vi "S2C_OM8257_Proc_SendCmd.vi"(7 "Local?":bool, 8 "Error In":errorcluster, 10 "Command":string, 11 "JSON String":string) -> (0 "Error Out":errorcluster, 3 "Response":variant)   [LabVIEW 2015]
uses:
  Uni-Therm/VIs/S2C_UNITHERM_Proc_Globals.vi
  S2C_OM8257_Proc_Globals.vi
  <instrlib>/Associated Research 82XX/Associated Research 82XX.lvlib
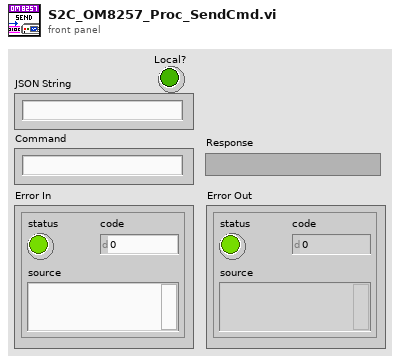
[diagram p1: front panel]
types:
  T1 = cluster{"Voltage (V)":u16, "High Limit Total (mA)":dbl, "Low Limit Total (mA)":dbl, "Ramp Up Time (s)":dbl, "Dwell Time (s)":dbl, "Arc Sense":u8, "Arc Detect":bool, "High Limit Real (mA)":dbl, "Low Limit Real (mA)":dbl, "Ramp Down Time (s)":dbl, "Continuity":bool, "Offset (mA)":dbl, "Auto Offset":bool, "DUT Output":bool, "Frequency (Hz)":u16, "Scanner?":bool, "Step Selection":i32, "Add Step":bool, "Scan1":i32, "Scan2":i32, "Scan3":i32, "Scan4":i32, "Scan5":i32, "Scan6":i32, "Scan7":i32, "Scan8":i32, "Scan9":i32, "Scan10":i32, "Scan11":i32, "Scan12":i32, "Scan13":i32, "Scan14":i32, "Scan15":i32, "Scan16":i32}
  T2 = cluster{"Scan1":i32, "Scan2":i32, "Scan3":i32, "Scan4":i32, "Scan5":i32, "Scan6":i32, "Scan7":i32, "Scan8":i32, "Scan9":i32, "Scan10":i32, "Scan11":i32, "Scan12":i32, "Scan13":i32, "Scan14":i32, "Scan15":i32, "Scan16":i32}
  T3 = cluster{"Voltage (1240V)":u16, "High Limit Total (10mA)":dbl, "Low Limit Total (0mA)":dbl, "Ramp Up Time (0.1s)":dbl, "Dwell Time (1s)":dbl, "Arc Sense (5)":u8, "Arc Detect (F: Off)":bool, "High Limit Real(10mA)":dbl, "Low Limit Real (0mA)":dbl, "Ramp Down Time (1s)":dbl, "Continuity (F: Off)":bool, "Offset (0mA)":dbl, "Auto Offset (F: Off)":bool, "DUT Output (F: Off)":bool, "Frequency (60Hz)":u16}
  T4 = cluster{"Leakage-Hi (V)":dbl, "Leakage-Lo (V)":dbl, "Voltage-Hi (V)":dbl, "Voltage-Lo (V)":dbl, "Dwell (s)":dbl, "Delay (s)":dbl, "Offset (uA)":dbl, "AC Src Voltage (V)":dbl, "AC Src A-Hi (A)":dbl, "AC Source":bool, "AC Src Frequency":dbl, "Auto Offset":bool, "Reverse":bool, "Active Link":bool, "AC Src OC Fold":bool, "Neutral":bool, "Ground":bool, "Leakage":bool, "Ranging Mode":bool, "AC Src Output":bool, "AC Src Range":bool, "Measure Device":u16, "Probe":u16, "Filter Mode":u16, "Scanner?":bool, "Step Selection":i32, "Add Step":bool, "Scan1":i32, "Scan2":i32, "Scan3":i32, "Scan4":i32, "Scan5":i32, "Scan6":i32, "Scan7":i32, "Scan8":i32, "Scan9":i32, "Scan10":i32, "Scan11":i32, "Scan12":i32, "Scan13":i32, "Scan14":i32, "Scan15":i32, "Scan16":i32}
  T5 = cluster{"Leakage-Hi (6000V)":dbl, "Leakage-Lo (0uA)":dbl, "Voltage-Hi (125V)":dbl, "Voltage-Lo (0V)":dbl, "Dwell (0.5s)":dbl, "Delay (1s)":dbl, "Offset  (0uA)":dbl, "AC Source Voltage (115V)":dbl, "AC Source A-Hi (0A)":dbl, "AC Source (F: OFF)":bool, "AC Source Frequency (60Hz)":dbl, "Auto Offset (F:OFF)":bool, "Reverse (F:OFF)":bool, "Active Link (F:OFF)":bool, "AC Source OC Fold (F:OFF)":bool, "Neutral (F:CLOSED)":bool, "Ground (F:CLOSED)":bool, "Leakage (F:RMS)":bool, "Ranging Mode (Auto)":bool, "AC Source Output (T:OPEN)":bool, "AC Source Range (F:LOW)":bool, "Measure Device (UL544NP)":u16, "Probe (Ground TO Line)":u16, "Filter Mode (AC+DC)":u16}
  T6 = cluster{"Current (25A)":dbl, "Voltage (8V)":dbl, "Hi-Limit (100mohm)":u16, "Lo-Limit (0mohm)":u16, "Dwell (1s)":dbl, "Offset (0mohm)":u16, "Auto Offset (OFF)":bool, "Frequency (60Hz)":u16, "DualCHEK (OFF)":u16}
  T7 = cluster{"Current (A)":dbl, "Voltage (V)":dbl, "Hi-Limit (mohm)":u16, "Lo-Limit (mhom)":u16, "Dwell (s)":dbl, "Offset (mhom)":u16, "Auto Offset":bool, "Frequency (Hz)":u16, "DualCHEK":u16, "Scanner Selection":i32, "Scanner?":bool, "Step Selection":i32, "Add Step":bool}
  T8 = cluster{"Voltage-Hi (125V)":dbl, "Voltage-Lo (0V)":dbl, "Amp-Hi (10A)":dbl, "Amp-Lo (0A)":dbl, "Dwell (1s)":dbl, "Delay (0.2s)":dbl, "Leakag-Hi (10mA)":dbl, "Leakage-Lo (0mA)":dbl, "Power-Hi (1000W)":u16, "Power-Lo (0W)":u16, "PF-Hi (1)":dbl, "PF-Lo (0)":dbl, "AC Source Voltage (115V)":dbl, "AC Source A-Hi (0A)":dbl, "AC Source (F: OFF)":bool, "AC Source Frequency (60Hz)":u16, "AC Source OC Fold (F:OFF)":bool, "AC Source Output (T:OPEN)":bool, "AC Source Range (F:LOW)":bool, "Active Link (F:OFF)":bool}
  T9 = cluster{"Voltage-Hi (V)":dbl, "Voltage-Lo (V)":dbl, "Amp-Hi (A)":dbl, "Amp-Lo (A)":dbl, "Dwell (s)":dbl, "Delay (s)":dbl, "Leakage-Hi (mA)":dbl, "Leakage-Lo (mA)":dbl, "Power-Hi (W)":u16, "Power-Lo (W)":u16, "PF-Lo":dbl, "PF-Hi":dbl, "AC Src Voltage (V)":dbl, "AC Src A-Hi (A)":dbl, "AC Source":bool, "AC Src Frequency (Hz)":u16, "AC Src OC Fold":bool, "AC Src Output":bool, "AC Src Range":bool, "Active Link":bool, "Step Selection":i32, "Add Step":bool}
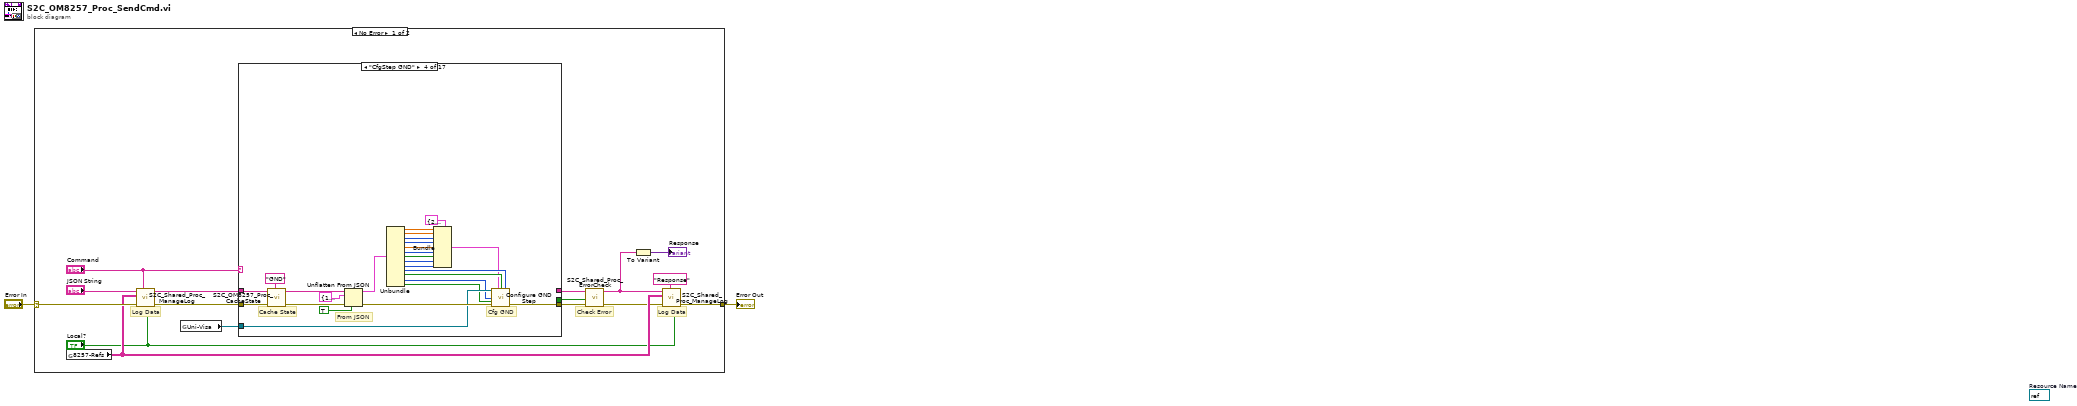
[diagram p0: block diagram]
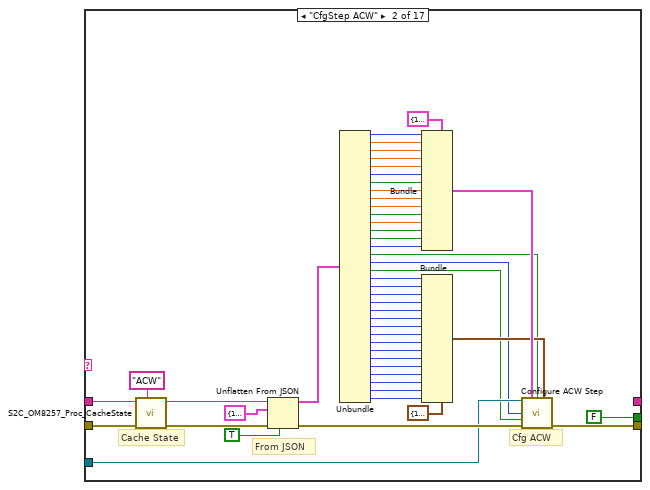
[diagram p3: hidden frame]
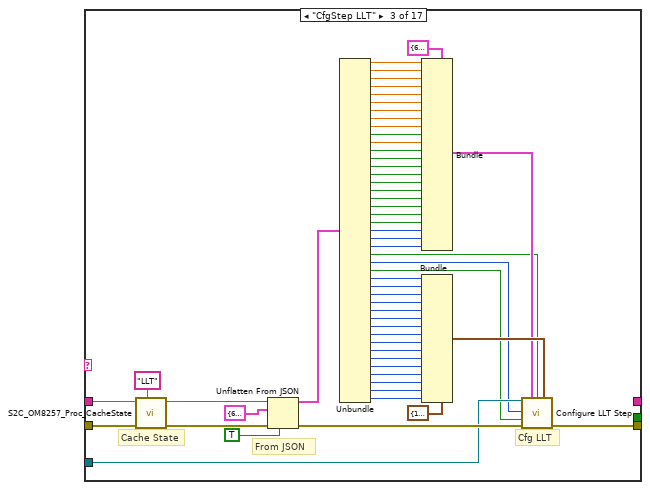
[diagram p4: hidden frame]
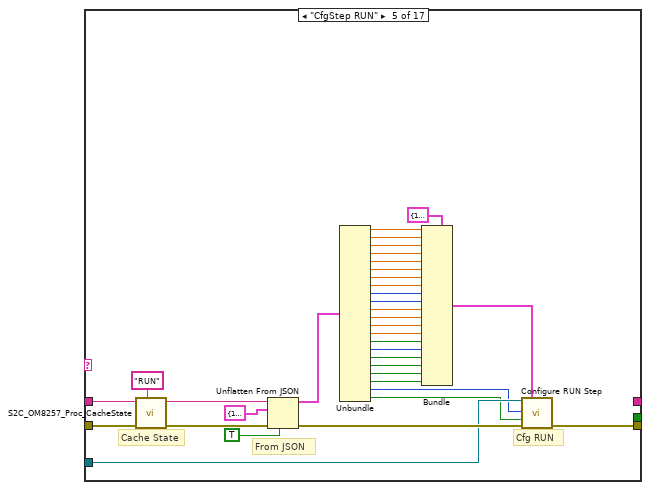
[diagram p5: hidden frame]
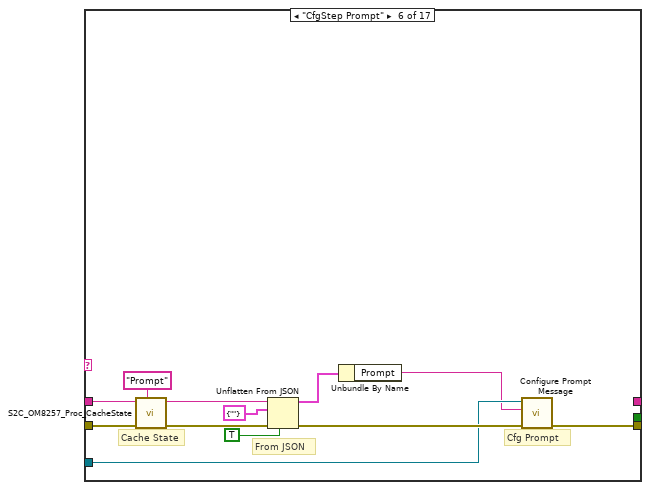
[diagram p6: hidden frame]
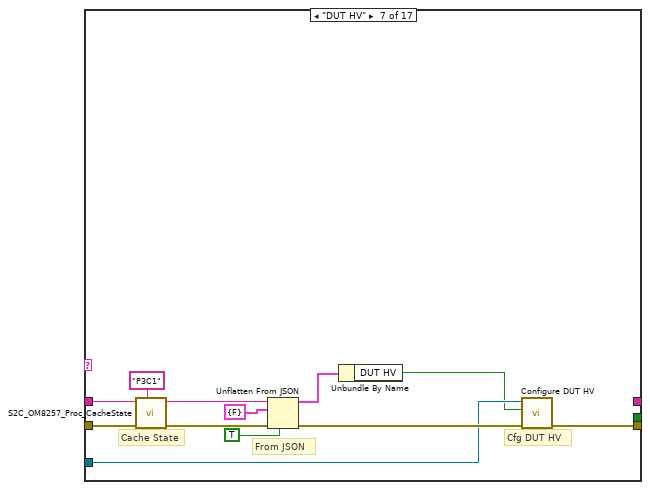
[diagram p7: hidden frame]
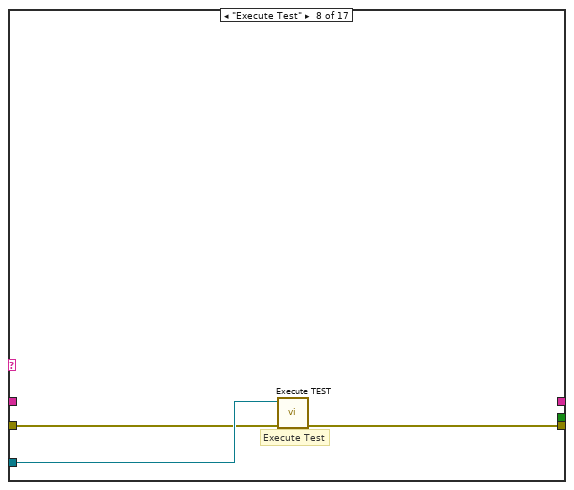
[diagram p8: hidden frame]
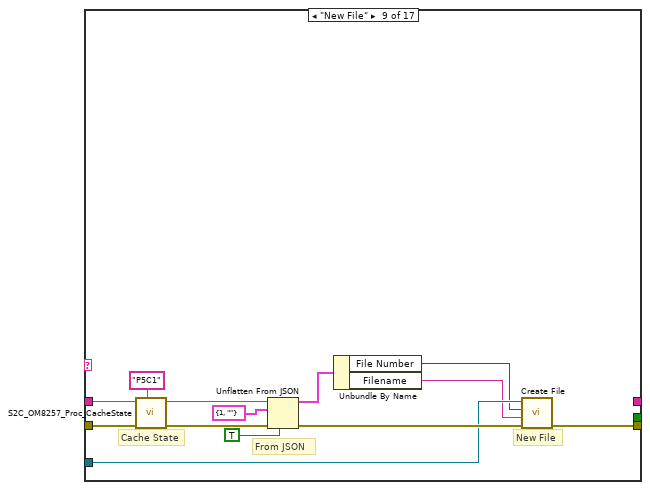
[diagram p9: hidden frame]
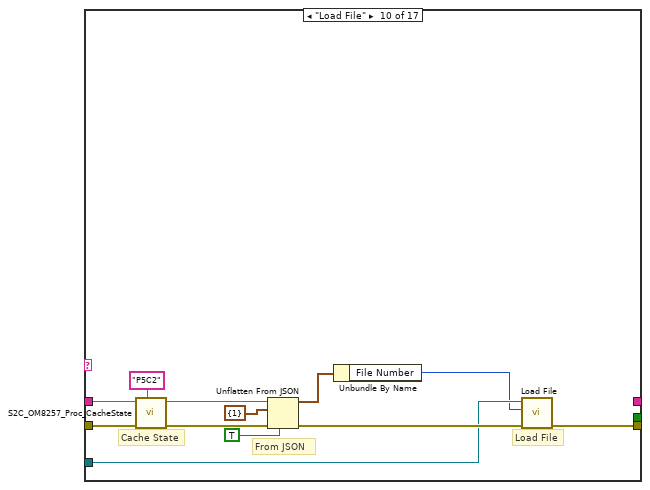
[diagram p10: hidden frame]
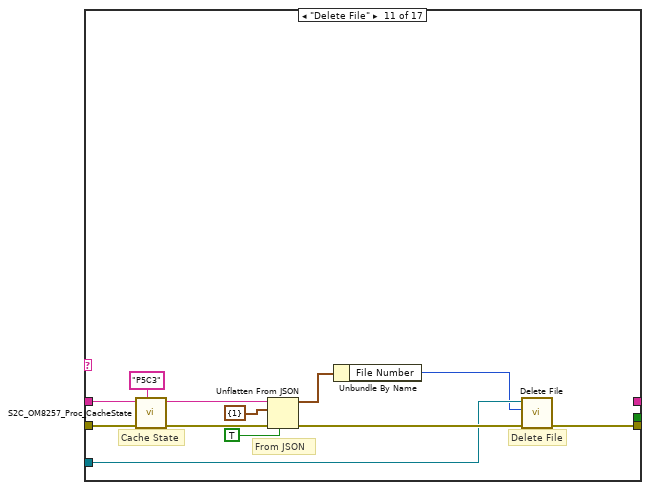
[diagram p11: hidden frame]
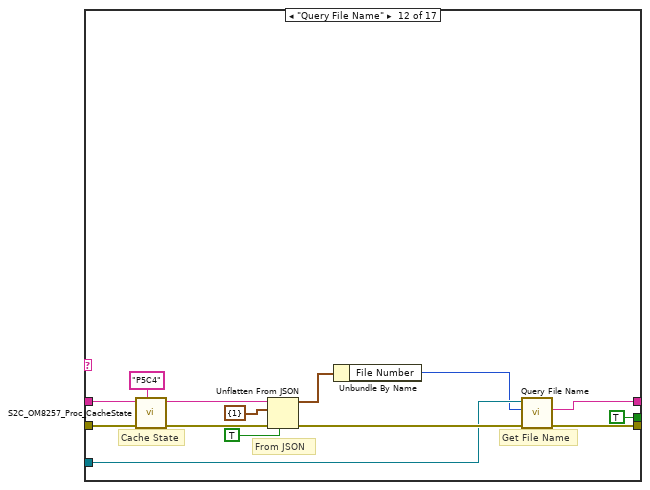
[diagram p12: hidden frame]
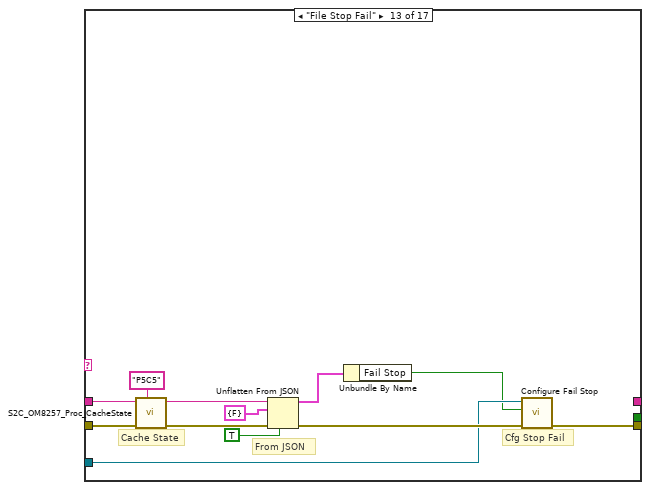
[diagram p13: hidden frame]
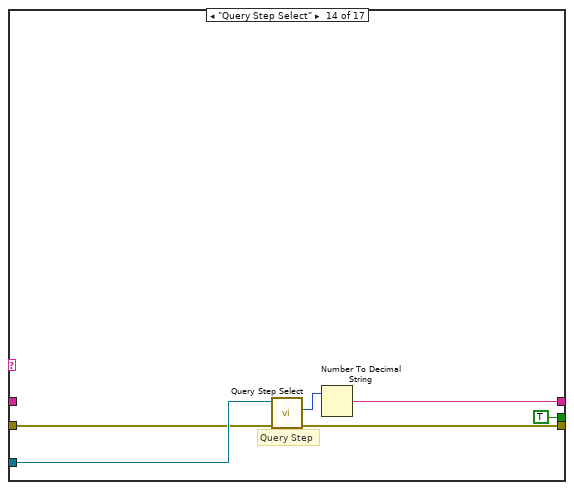
[diagram p14: hidden frame]
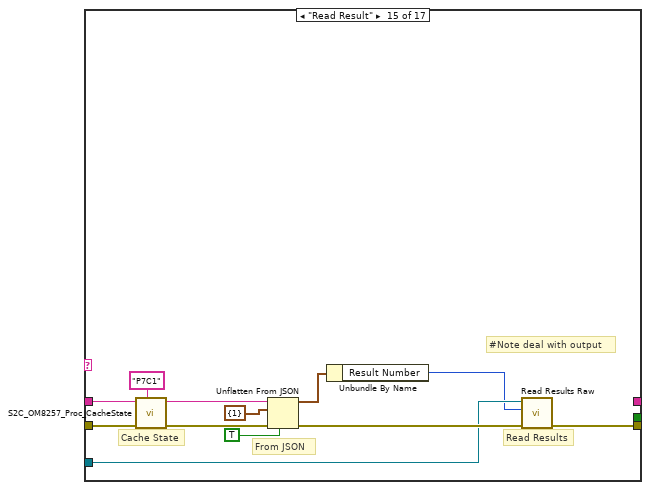
[diagram p15: hidden frame]
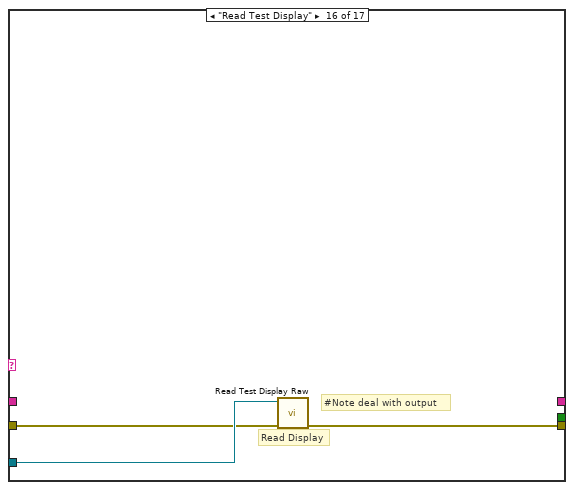
[diagram p16: hidden frame]
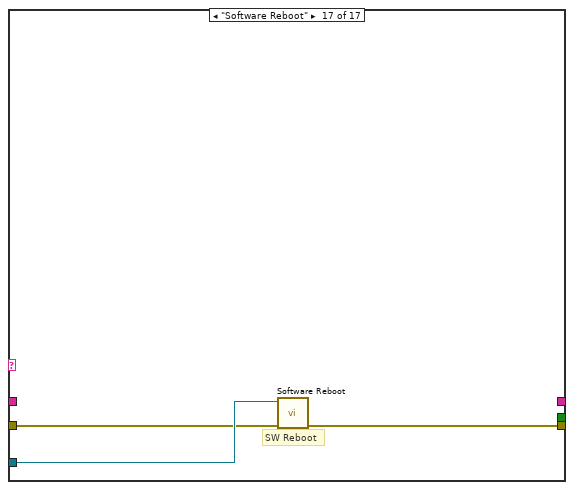
[diagram p17: hidden frame]
diagram:
  (unwired) refnum<visa-resource-name> refnum  # Resource Name
  n1 = case shown="No Error" "Error In" {
    selector: "Error In" -> [w17 w303]
    tunnel: [w16 w303] -> w1
    frame No Error {
      # "Check Error"
      # "Log Data"
      # "Log Data"
      n2 = global read "S2C_OM8257_Proc_Globals.vi" "8257-Refs"() -> (w14:string[][])
      n3 = call "S2C_Shared_Proc_ManageLog.vi"("Local?"="Local?", "Command"="Command", "Error In"=w17, "Refs"=w14, "Data In"="JSON String") -> ("Error Out"=w8:errorcluster, "Data Out"=w7:string)  [unwired: 5 in]
      n4 = global read "S2C_UNITHERM_Proc_Globals.vi" "Uni-Visa"() -> (w6:refnum<visa-resource-name>)
      n5 = case shown="\"CfgStep GND\"" "Command" {
        tunnel: [w19 w67 w125 w151 w186 w198 w210 w215 w226 w238 w250 w264 w276 w284 w294 w299 w302] -> w13
        tunnel: w8 -> [w19 w65 w123 w149 w184 w196 w208 w213 w224 w236 w248 w262 w274 w282 w292 w297 w300]
        tunnel: w7 -> [_ w64 w122 w148 w183 w195 w207 _ w223 w235 w247 w261 w273 _ w291 _ _]
        tunnel: w6 -> [_ w59 w119 w145 w180 w192 w204 w214 w220 w232 w244 w258 w270 w283 w288 w298 w301]
        tunnel: [_ FALSE ("ExpReply?") _ _ _ _ _ _ _ _ _ TRUE ("ExpReply?") _ TRUE ("ExpReply?") _ _ _] -> w5
        tunnel: [_ _ _ _ _ _ _ _ _ _ _ w254 _ w281 _ _ _] -> w3
        frame "Other", Default {
        }
        frame "CfgStep ACW" {
          # "Cache State"
          # "Cfg ACW"
          # "From JSON"
          n6 = call "S2C_OM8257_Proc_CacheState.vi"("Label"="ACW", "Error In"=w65, "Data In"=w64) -> ("Error Out"=w63:errorcluster, "Data Out"=w62:string)  [unwired: 7 in]
          n7 = Unflatten From JSON(JSON string=w62, type and defaults=T1 {"Voltage (V)"=1240, "High Limit Total (mA)"=10.0, "Low Limit Total (mA)"=0.0, "Ramp Up Time (s)"=0.1, "Dwell Time (s)"=1.0, "Arc Sense"=5, "Arc Detect"=FALSE, "High Limit Real (mA)"=10.0, "Low Limit Real (mA)"=0.0, "Ramp Down Time (s)"=0.0, "Continuity"=FALSE, "Offset (mA)"=0.0, "Auto Offset"=FALSE, "DUT Output"=FALSE, "Frequency (Hz)"=60, "Scanner?"=FALSE, "Step Selection"=1, "Add Step"=FALSE, "Scan1"=1, "Scan2"=1, "Scan3"=1, "Scan4"=1, "Scan5"=1, "Scan6"=1, "Scan7"=1, "Scan8"=1, "Scan9"=1, "Scan10"=1, "Scan11"=1, "Scan12"=1, "Scan13"=1, "Scan14"=1, "Scan15"=1, "Scan16"=1} ("ACW"), default null elements? (F)=TRUE, error in (no error)=w63) -> (value=w39:T1, error out=w68:errorcluster)  [unwired: 3 in]
          n8 = Unbundle(w39) -> ("Voltage (V)"=w34:u16, "High Limit Total (mA)"=w33:dbl, "Low Limit Total (mA)"=w32:dbl, "Ramp Up Time (s)"=w31:dbl, "Dwell Time (s)"=w30:dbl, "Arc Sense"=w29:u8, "Arc Detect"=w28:bool, "High Limit Real (mA)"=w27:dbl, "Low Limit Real (mA)"=w26:dbl, "Ramp Down Time (s)"=w25:dbl, "Continuity"=w24:bool, "Offset (mA)"=w23:dbl, "Auto Offset"=w22:bool, "DUT Output"=w21:bool, "Frequency (Hz)"=w20:u16, "Scanner?"=w38:bool, "Step Selection"=w37:i32, "Add Step"=w36:bool, "Scan1"=w57:i32, "Scan2"=w56:i32, "Scan3"=w55:i32, "Scan4"=w54:i32, "Scan5"=w53:i32, "Scan6"=w52:i32, "Scan7"=w51:i32, "Scan8"=w50:i32, "Scan9"=w49:i32, "Scan10"=w48:i32, "Scan11"=w47:i32, "Scan12"=w46:i32, "Scan13"=w45:i32, "Scan14"=w44:i32, "Scan15"=w43:i32, "Scan16"=w42:i32)
          n9 = Bundle(cluster=T3 {"Voltage (1240V)"=1240, "High Limit Total (10mA)"=10.0, "Low Limit Total (0mA)"=0.0, "Ramp Up Time (0.1s)"=0.1, "Dwell Time (1s)"=1.0, "Arc Sense (5)"=5, "Arc Detect (F: Off)"=FALSE, "High Limit Real(10mA)"=10.0, "Low Limit Real (0mA)"=0.0, "Ramp Down Time (1s)"=0.0, "Continuity (F: Off)"=FALSE, "Offset (0mA)"=0.0, "Auto Offset (F: Off)"=FALSE, "DUT Output (F: Off)"=FALSE, "Frequency (60Hz)"=60} ("ACW Test Parameters in"), "Voltage (1240V)"=w34, "High Limit Total (10mA)"=w33, "Low Limit Total (0mA)"=w32, "Ramp Up Time (0.1s)"=w31, "Dwell Time (1s)"=w30, "Arc Sense (5)"=w29, "Arc Detect (F: Off)"=w28, "High Limit Real(10mA)"=w27, "Low Limit Real (0mA)"=w26, "Ramp Down Time (1s)"=w25, "Continuity (F: Off)"=w24, "Offset (0mA)"=w23, "Auto Offset (F: Off)"=w22, "DUT Output (F: Off)"=w21, "Frequency (60Hz)"=w20) -> (w60:T3)
          n10 = Bundle(cluster=T2 {"Scan1"=1, "Scan2"=1, "Scan3"=1, "Scan4"=1, "Scan5"=1, "Scan6"=1, "Scan7"=1, "Scan8"=1, "Scan9"=1, "Scan10"=1, "Scan11"=1, "Scan12"=1, "Scan13"=1, "Scan14"=1, "Scan15"=1, "Scan16"=1} ("Scanner Settings in"), "Scan1"=w57, "Scan2"=w56, "Scan3"=w55, "Scan4"=w54, "Scan5"=w53, "Scan6"=w52, "Scan7"=w51, "Scan8"=w50, "Scan9"=w49, "Scan10"=w48, "Scan11"=w47, "Scan12"=w46, "Scan13"=w45, "Scan14"=w44, "Scan15"=w43, "Scan16"=w42) -> (w40:T2)
          n11 = call <instrlib>:"Configure ACW Step.vi"("VISA resource name"=w59, "ACW Test Parameters in"=w60, "Scanner? (F: No)"=w38, "Scanner Settings in"=w40, "Step Selection (1)"=w37, "Add Step (Edit)"=w36, "error in (no error)"=w68) -> ("error out"=w67:errorcluster)  [unwired: 7 in, 1 out]
        }
        frame "CfgStep LLT" {
          # "Cache State"
          # "Cfg LLT"
          # "From JSON"
          n12 = call "S2C_OM8257_Proc_CacheState.vi"("Label"="LLT", "Error In"=w123, "Data In"=w122) -> ("Error Out"=w121:errorcluster, "Data Out"=w120:string)  [unwired: 7 in]
          n13 = Unflatten From JSON(JSON string=w120, type and defaults=T4 {"Leakage-Hi (V)"=6000.0, "Leakage-Lo (V)"=0.0, "Voltage-Hi (V)"=125.0, "Voltage-Lo (V)"=0.0, "Dwell (s)"=0.5, "Delay (s)"=1.0, "Offset (uA)"=10.0, "AC Src Voltage (V)"=115.0, "AC Src A-Hi (A)"=0.0, "AC Source"=FALSE, "AC Src Frequency"=60.0, "Auto Offset"=FALSE, "Reverse"=FALSE, "Active Link"=FALSE, "AC Src OC Fold"=FALSE, "Neutral"=FALSE, "Ground"=FALSE, "Leakage"=FALSE, "Ranging Mode"=FALSE, "AC Src Output"=TRUE, "AC Src Range"=TRUE, "Measure Device"=0, "Probe"=0, "Filter Mode"=0, "Scanner?"=FALSE, "Step Selection"=1, "Add Step"=FALSE, "Scan1"=1, "Scan2"=1, "Scan3"=1, "Scan4"=1, "Scan5"=1, "Scan6"=1, "Scan7"=1, "Scan8"=1, "Scan9"=1, "Scan10"=1, "Scan11"=1, "Scan12"=1, "Scan13"=1, "Scan14"=1, "Scan15"=1, "Scan16"=1} ("LLT"), default null elements? (F)=TRUE, error in (no error)=w121) -> (value=w116:T4, error out=w126:errorcluster)  [unwired: 3 in]
          n14 = Unbundle(w116) -> ("Leakage-Hi (V)"=w70:dbl, "Leakage-Lo (V)"=w71:dbl, "Voltage-Hi (V)"=w72:dbl, "Voltage-Lo (V)"=w73:dbl, "Dwell (s)"=w74:dbl, "Delay (s)"=w75:dbl, "Offset (uA)"=w76:dbl, "AC Src Voltage (V)"=w77:dbl, "AC Src A-Hi (A)"=w78:dbl, "AC Source"=w79:bool, "AC Src Frequency"=w80:dbl, "Auto Offset"=w81:bool, "Reverse"=w82:bool, "Active Link"=w83:bool, "AC Src OC Fold"=w84:bool, "Neutral"=w85:bool, "Ground"=w86:bool, "Leakage"=w87:bool, "Ranging Mode"=w88:bool, "AC Src Output"=w89:bool, "AC Src Range"=w90:bool, "Measure Device"=w91:u16, "Probe"=w92:u16, "Filter Mode"=w93:u16, "Scanner?"=w94:bool, "Step Selection"=w95:i32, "Add Step"=w96:bool, "Scan1"=w97:i32, "Scan2"=w98:i32, "Scan3"=w99:i32, "Scan4"=w100:i32, "Scan5"=w101:i32, "Scan6"=w102:i32, "Scan7"=w103:i32, "Scan8"=w104:i32, "Scan9"=w105:i32, "Scan10"=w106:i32, "Scan11"=w107:i32, "Scan12"=w108:i32, "Scan13"=w109:i32, "Scan14"=w110:i32, "Scan15"=w111:i32, "Scan16"=w112:i32)
          n15 = Bundle(cluster=T5 {"Leakage-Hi (6000V)"=6000.0, "Leakage-Lo (0uA)"=0.0, "Voltage-Hi (125V)"=125.0, "Voltage-Lo (0V)"=0.0, "Dwell (0.5s)"=0.5, "Delay (1s)"=1.0, "Offset  (0uA)"=0.0, "AC Source Voltage (115V)"=115.0, "AC Source A-Hi (0A)"=0.0, "AC Source (F: OFF)"=FALSE, "AC Source Frequency (60Hz)"=60.0, "Auto Offset (F:OFF)"=FALSE, "Reverse (F:OFF)"=FALSE, "Active Link (F:OFF)"=FALSE, "AC Source OC Fold (F:OFF)"=FALSE, "Neutral (F:CLOSED)"=FALSE, "Ground (F:CLOSED)"=FALSE, "Leakage (F:RMS)"=FALSE, "Ranging Mode (Auto)"=FALSE, "AC Source Output (T:OPEN)"=TRUE, "AC Source Range (F:LOW)"=TRUE, "Measure Device (UL544NP)"=0, "Probe (Ground TO Line)"=0, "Filter Mode (AC+DC)"=0} ("LLT Test Parameters in"), "Leakage-Hi (6000V)"=w70, "Leakage-Lo (0uA)"=w71, "Voltage-Hi (125V)"=w72, "Voltage-Lo (0V)"=w73, "Dwell (0.5s)"=w74, "Delay (1s)"=w75, "Offset  (0uA)"=w76, "AC Source Voltage (115V)"=w77, "AC Source A-Hi (0A)"=w78, "AC Source (F: OFF)"=w79, "AC Source Frequency (60Hz)"=w80, "Auto Offset (F:OFF)"=w81, "Reverse (F:OFF)"=w82, "Active Link (F:OFF)"=w83, "AC Source OC Fold (F:OFF)"=w84, "Neutral (F:CLOSED)"=w85, "Ground (F:CLOSED)"=w86, "Leakage (F:RMS)"=w87, "Ranging Mode (Auto)"=w88, "AC Source Output (T:OPEN)"=w89, "AC Source Range (F:LOW)"=w90, "Measure Device (UL544NP)"=w91, "Probe (Ground TO Line)"=w92, "Filter Mode (AC+DC)"=w93) -> (w114:T5)
          n16 = Bundle(cluster=T2 {"Scan1"=1, "Scan2"=1, "Scan3"=1, "Scan4"=1, "Scan5"=1, "Scan6"=1, "Scan7"=1, "Scan8"=1, "Scan9"=1, "Scan10"=1, "Scan11"=1, "Scan12"=1, "Scan13"=1, "Scan14"=1, "Scan15"=1, "Scan16"=1} ("Scanner Settings in"), "Scan1"=w97, "Scan2"=w98, "Scan3"=w99, "Scan4"=w100, "Scan5"=w101, "Scan6"=w102, "Scan7"=w103, "Scan8"=w104, "Scan9"=w105, "Scan10"=w106, "Scan11"=w107, "Scan12"=w108, "Scan13"=w109, "Scan14"=w110, "Scan15"=w111, "Scan16"=w112) -> (w117:T2)
          n17 = call <instrlib>:"Configure LLT Step.vi"("VISA resource name"=w119, "LLT Test Parameters in"=w114, "Scanner? (F:OFF)"=w94, "Scanner Settings in"=w117, "Step Selection (1)"=w95, "Add Step (Edit)"=w96, "error in (no error)"=w126) -> ("error out"=w125:errorcluster)  [unwired: 7 in, 1 out]
        }
        frame "CfgStep GND" {
          # "Cache State"
          # "Cfg GND"
          # "From JSON"
          n18 = call "S2C_OM8257_Proc_CacheState.vi"("Label"="GND", "Error In"=w149, "Data In"=w148) -> ("Error Out"=w147:errorcluster, "Data Out"=w146:string)  [unwired: 7 in]
          n19 = Unflatten From JSON(JSON string=w146, type and defaults=T7 {"Current (A)"=1240.0, "Voltage (V)"=10.0, "Hi-Limit (mohm)"=100, "Lo-Limit (mhom)"=0, "Dwell (s)"=1.0, "Offset (mhom)"=0, "Auto Offset"=FALSE, "Frequency (Hz)"=60, "DualCHEK"=0, "Scanner Selection"=0, "Scanner?"=FALSE, "Step Selection"=1, "Add Step"=FALSE} ("GND"), default null elements? (F)=TRUE, error in (no error)=w147) -> (value=w144:T7, error out=w152:errorcluster)  [unwired: 3 in]
          n20 = Unbundle(w144) -> ("Current (A)"=w135:dbl, "Voltage (V)"=w136:dbl, "Hi-Limit (mohm)"=w137:u16, "Lo-Limit (mhom)"=w138:u16, "Dwell (s)"=w139:dbl, "Offset (mhom)"=w140:u16, "Auto Offset"=w141:bool, "Frequency (Hz)"=w142:u16, "DualCHEK"=w143:u16, "Scanner Selection"=w132:i32, "Scanner?"=w131:bool, "Step Selection"=w129:i32, "Add Step"=w128:bool)
          n21 = Bundle(cluster=T6 {"Current (25A)"=25.0, "Voltage (8V)"=8.0, "Hi-Limit (100mohm)"=100, "Lo-Limit (0mohm)"=0, "Dwell (1s)"=1.0, "Offset (0mohm)"=0, "Auto Offset (OFF)"=FALSE, "Frequency (60Hz)"=60, "DualCHEK (OFF)"=0} ("GND Test Parameters in"), "Current (25A)"=w135, "Voltage (8V)"=w136, "Hi-Limit (100mohm)"=w137, "Lo-Limit (0mohm)"=w138, "Dwell (1s)"=w139, "Offset (0mohm)"=w140, "Auto Offset (OFF)"=w141, "Frequency (60Hz)"=w142, "DualCHEK (OFF)"=w143) -> (w130:T6)
          n22 = call <instrlib>:"Configure GND Step.vi"("VISA resource name"=w145, "GND Test Parameters in"=w130, "Scanner? (F:No)"=w131, "Scanner Selection (0:None)"=w132, "Step Selection (1)"=w129, "Add Step (Edit)"=w128, "error in (no error)"=w152) -> ("error out"=w151:errorcluster)  [unwired: 7 in, 1 out]
        }
        frame "CfgStep RUN" {
          # "Cache State"
          # "Cfg RUN"
          # "From JSON"
          n23 = call "S2C_OM8257_Proc_CacheState.vi"("Label"="RUN", "Error In"=w184, "Data In"=w183) -> ("Error Out"=w182:errorcluster, "Data Out"=w181:string)  [unwired: 7 in]
          n24 = Unflatten From JSON(JSON string=w181, type and defaults=T9 {"Voltage-Hi (V)"=125.0, "Voltage-Lo (V)"=0.0, "Amp-Hi (A)"=10.0, "Amp-Lo (A)"=0.0, "Dwell (s)"=1.0, "Delay (s)"=0.2, "Leakage-Hi (mA)"=10.0, "Leakage-Lo (mA)"=0.0, "Power-Hi (W)"=1000, "Power-Lo (W)"=0, "PF-Lo"=0.0, "PF-Hi"=1.0, "AC Src Voltage (V)"=115.0, "AC Src A-Hi (A)"=0.0, "AC Source"=FALSE, "AC Src Frequency (Hz)"=60, "AC Src OC Fold"=FALSE, "AC Src Output"=TRUE, "AC Src Range"=TRUE, "Active Link"=FALSE, "Step Selection"=1, "Add Step"=FALSE} ("RUN"), default null elements? (F)=TRUE, error in (no error)=w182) -> (value=w179:T9, error out=w187:errorcluster)  [unwired: 3 in]
          n25 = Unbundle(w179) -> ("Voltage-Hi (V)"=w159:dbl, "Voltage-Lo (V)"=w160:dbl, "Amp-Hi (A)"=w161:dbl, "Amp-Lo (A)"=w162:dbl, "Dwell (s)"=w163:dbl, "Delay (s)"=w164:dbl, "Leakage-Hi (mA)"=w165:dbl, "Leakage-Lo (mA)"=w166:dbl, "Power-Hi (W)"=w167:u16, "Power-Lo (W)"=w168:u16, "PF-Lo"=w169:dbl, "PF-Hi"=w170:dbl, "AC Src Voltage (V)"=w171:dbl, "AC Src A-Hi (A)"=w172:dbl, "AC Source"=w173:bool, "AC Src Frequency (Hz)"=w174:u16, "AC Src OC Fold"=w175:bool, "AC Src Output"=w176:bool, "AC Src Range"=w177:bool, "Active Link"=w178:bool, "Step Selection"=w156:i32, "Add Step"=w155:bool)
          n26 = Bundle(cluster=T8 {"Voltage-Hi (125V)"=125.0, "Voltage-Lo (0V)"=0.0, "Amp-Hi (10A)"=10.0, "Amp-Lo (0A)"=0.0, "Dwell (1s)"=1.0, "Delay (0.2s)"=0.2, "Leakag-Hi (10mA)"=10.0, "Leakage-Lo (0mA)"=0.0, "Power-Hi (1000W)"=1000, "Power-Lo (0W)"=0, "PF-Hi (1)"=1.0, "PF-Lo (0)"=0.0, "AC Source Voltage (115V)"=115.0, "AC Source A-Hi (0A)"=0.0, "AC Source (F: OFF)"=FALSE, "AC Source Frequency (60Hz)"=60, "AC Source OC Fold (F:OFF)"=FALSE, "AC Source Output (T:OPEN)"=TRUE, "AC Source Range (F:LOW)"=TRUE, "Active Link (F:OFF)"=TRUE} ("Run Test Parameters in"), "Voltage-Hi (125V)"=w159, "Voltage-Lo (0V)"=w160, "Amp-Hi (10A)"=w161, "Amp-Lo (0A)"=w162, "Dwell (1s)"=w163, "Delay (0.2s)"=w164, "Leakag-Hi (10mA)"=w165, "Leakage-Lo (0mA)"=w166, "Power-Hi (1000W)"=w167, "Power-Lo (0W)"=w168, "PF-Hi (1)"=w169, "PF-Lo (0)"=w170, "AC Source Voltage (115V)"=w171, "AC Source A-Hi (0A)"=w172, "AC Source (F: OFF)"=w173, "AC Source Frequency (60Hz)"=w174, "AC Source OC Fold (F:OFF)"=w175, "AC Source Output (T:OPEN)"=w176, "AC Source Range (F:LOW)"=w177, "Active Link (F:OFF)"=w178) -> (w154:T8)
          n27 = call <instrlib>:"Configure RUN Step.vi"("VISA resource name"=w180, "Run Test Parameters in"=w154, "Step Selection (1)"=w156, "Add Step (Edit)"=w155, "error in (no error)"=w187) -> ("error out"=w186:errorcluster)  [unwired: 9 in, 1 out]
        }
        frame "CfgStep Prompt" {
          # "Cache State"
          # "Cfg Prompt"
          # "From JSON"
          n28 = call "S2C_OM8257_Proc_CacheState.vi"("Label"="Prompt", "Error In"=w196, "Data In"=w195) -> ("Error Out"=w194:errorcluster, "Data Out"=w193:string)  [unwired: 7 in]
          n29 = Unflatten From JSON(JSON string=w193, type and defaults=cluster{"Prompt":string} {"Prompt"=""} ("Prompt"), default null elements? (F)=TRUE, error in (no error)=w194) -> (value=w191:cluster{"Prompt":string}, error out=w199:errorcluster)  [unwired: 3 in]
          n30 = Unbundle By Name(w191) -> ("Prompt"=w189:string)
          n31 = call <instrlib>:"Configure Prompt Message.vi"("error in (no error)"=w199, "Prompt (empty)"=w189, "VISA resource name"=w192) -> ("error out"=w198:errorcluster)  [unwired: 7 in, 1 out]
        }
        frame "DUT HV" {
          # "Cache State"
          # "Cfg DUT HV"
          # "From JSON"
          n32 = call "S2C_OM8257_Proc_CacheState.vi"("Label"="P3C1", "Error In"=w208, "Data In"=w207) -> ("Error Out"=w206:errorcluster, "Data Out"=w205:string)  [unwired: 7 in]
          n33 = Unflatten From JSON(JSON string=w205, type and defaults=cluster{"DUT HV":bool} {"DUT HV"=FALSE} ("P3C1"), default null elements? (F)=TRUE, error in (no error)=w206) -> (value=w203:cluster{"DUT HV":bool}, error out=w211:errorcluster)  [unwired: 3 in]
          n34 = Unbundle By Name(w203) -> ("DUT HV"=w201:bool)
          n35 = call <instrlib>:"Configure DUT HV.vi"("error in (no error)"=w211, "DUT HV (F:OFF)"=w201, "VISA resource name"=w204) -> ("error out"=w210:errorcluster)  [unwired: 7 in, 1 out]
        }
        frame "Execute Test" {
          # "Execute Test"
          n36 = call <instrlib>:"Execute TEST.vi"("error in (no error)"=w213, "VISA resource name"=w214) -> ("error out"=w215:errorcluster)  [unwired: 8 in, 1 out]
        }
        frame "New File" {
          # "Cache State"
          # "New File"
          # "From JSON"
          n37 = call "S2C_OM8257_Proc_CacheState.vi"("Label"="P5C1", "Error In"=w224, "Data In"=w223) -> ("Error Out"=w222:errorcluster, "Data Out"=w221:string)  [unwired: 7 in]
          n38 = Unflatten From JSON(JSON string=w221, type and defaults=cluster{"File Number":i32, "Filename":string} {"File Number"=1, "Filename"=""} ("P5C1"), default null elements? (F)=TRUE, error in (no error)=w222) -> (value=w219:cluster{"File Number":i32, "Filename":string}, error out=w227:errorcluster)  [unwired: 3 in]
          n39 = Unbundle By Name(w219) -> ("File Number"=w218:i32, "Filename"=w217:string)
          n40 = call <instrlib>:"Create File.vi"("error in (no error)"=w227, "File Name (Temp)"=w217, "File Number (1)"=w218, "VISA resource name"=w220) -> ("error out"=w226:errorcluster)  [unwired: 6 in, 1 out]
        }
        frame "Load File" {
          # "Cache State"
          # "Load File"
          # "From JSON"
          n41 = call "S2C_OM8257_Proc_CacheState.vi"("Label"="P5C2", "Error In"=w236, "Data In"=w235) -> ("Error Out"=w234:errorcluster, "Data Out"=w233:string)  [unwired: 7 in]
          n42 = Unflatten From JSON(JSON string=w233, type and defaults=cluster{"File Number":u16} {"File Number"=1} ("P5C2"), default null elements? (F)=TRUE, error in (no error)=w234) -> (value=w231:cluster{"File Number":u16}, error out=w239:errorcluster)  [unwired: 3 in]
          n43 = Unbundle By Name(w231) -> ("File Number"=w230:u16)
          n44 = call <instrlib>:"Load File.vi"("error in (no error)"=w239, "File Number (1)"=w230, "VISA resource name"=w232) -> ("error out"=w238:errorcluster)  [unwired: 7 in, 1 out]
        }
        frame "Delete File" {
          # "Cache State"
          # "Delete File"
          # "From JSON"
          n45 = call "S2C_OM8257_Proc_CacheState.vi"("Label"="P5C3", "Error In"=w248, "Data In"=w247) -> ("Error Out"=w246:errorcluster, "Data Out"=w245:string)  [unwired: 7 in]
          n46 = Unflatten From JSON(JSON string=w245, type and defaults=cluster{"File Number":u16} {"File Number"=1} ("P5C2"), default null elements? (F)=TRUE, error in (no error)=w246) -> (value=w243:cluster{"File Number":u16}, error out=w251:errorcluster)  [unwired: 3 in]
          n47 = Unbundle By Name(w243) -> ("File Number"=w242:u16)
          n48 = call <instrlib>:"Delete File.vi"("error in (no error)"=w251, "File Number (1)"=w242, "VISA resource name"=w244) -> ("error out"=w250:errorcluster)  [unwired: 7 in, 1 out]
        }
        frame "Query File Name" {
          # "Cache State"
          # "Get File Name"
          # "From JSON"
          n49 = call "S2C_OM8257_Proc_CacheState.vi"("Label"="P5C4", "Error In"=w262, "Data In"=w261) -> ("Error Out"=w260:errorcluster, "Data Out"=w259:string)  [unwired: 7 in]
          n50 = Unflatten From JSON(JSON string=w259, type and defaults=cluster{"File Number":u16} {"File Number"=1} ("P5C2"), default null elements? (F)=TRUE, error in (no error)=w260) -> (value=w257:cluster{"File Number":u16}, error out=w265:errorcluster)  [unwired: 3 in]
          n51 = Unbundle By Name(w257) -> ("File Number"=w256:u16)
          n52 = call <instrlib>:"Query File Name.vi"("error in (no error)"=w265, "File Number (1)"=w256, "VISA resource name"=w258) -> ("error out"=w264:errorcluster, "File Name"=w254:string)  [unwired: 6 in, 1 out]
        }
        frame "File Stop Fail" {
          # "Cache State"
          # "Cfg Stop Fail"
          # "From JSON"
          n53 = call "S2C_OM8257_Proc_CacheState.vi"("Label"="P5C5", "Error In"=w274, "Data In"=w273) -> ("Error Out"=w272:errorcluster, "Data Out"=w271:string)  [unwired: 7 in]
          n54 = Unflatten From JSON(JSON string=w271, type and defaults=cluster{"Fail Stop":bool} {"Fail Stop"=FALSE} ("P5C5"), default null elements? (F)=TRUE, error in (no error)=w272) -> (value=w269:cluster{"Fail Stop":bool}, error out=w277:errorcluster)  [unwired: 3 in]
          n55 = Unbundle By Name(w269) -> ("Fail Stop"=w267:bool)
          n56 = call <instrlib>:"Configure Fail Stop.vi"("error in (no error)"=w277, "Fail Stop (F:Off)"=w267, "VISA resource name"=w270) -> ("error out"=w276:errorcluster)  [unwired: 7 in, 1 out]
        }
        frame "Query Step Select" {
          # "Query Step"
          n57 = call <instrlib>:"Query Step Select.vi"("error in (no error)"=w282, "VISA resource name"=w283) -> ("error out"=w284:errorcluster, "Step Number"=w280:i32)  [unwired: 7 in, 1 out]
          n58 = Number To Decimal String(number=w280) -> (decimal integer string=w281:string)  [unwired: 1 in]
        }
        frame "Read Result" {
          # "#Note deal with output"
          # "Cache State"
          # "Read Results"
          # "From JSON"
          n59 = call "S2C_OM8257_Proc_CacheState.vi"("Label"="P7C1", "Error In"=w292, "Data In"=w291) -> ("Error Out"=w290:errorcluster, "Data Out"=w289:string)  [unwired: 7 in]
          n60 = Unflatten From JSON(JSON string=w289, type and defaults=cluster{"Result Number":i32} {"Result Number"=1} ("P7C1"), default null elements? (F)=TRUE, error in (no error)=w290) -> (value=w287:cluster{"Result Number":i32}, error out=w295:errorcluster)  [unwired: 3 in]
          n61 = Unbundle By Name(w287) -> ("Result Number"=w286:i32)
          n62 = call <instrlib>:"Read Results Raw.vi"("error in (no error)"=w295, "Buffer number (1)"=w286, "VISA resource name"=w288) -> ("error out"=w294:errorcluster)  [unwired: 6 in, 2 out]
        }
        frame "Read Test Display" {
          # "#Note deal with output"
          # "Read Display"
          n63 = call <instrlib>:"Read Test Display Raw.vi"("error in (no error)"=w297, "VISA resource name"=w298) -> ("error out"=w299:errorcluster)  [unwired: 7 in, 2 out]
        }
        frame "Software Reboot" {
          # "SW Reboot"
          n64 = call <instrlib>:"Software Reboot.vi"("error in (no error)"=w300, "VISA resource name"=w301) -> ("error out"=w302:errorcluster)  [unwired: 8 in, 1 out]
        }
      }
      n65 = call "S2C_Shared_Proc_ErrorCheck.vi"("Error In"=w13, "ExpReply?"=w5, "Reply Text"=w3) -> ("Error Out"=w12:errorcluster, "Status"=w10:string)  [unwired: 7 in]
      n66 = To Variant(anything=w10) -> (Variant=→"Response":variant)
      n67 = call "S2C_Shared_Proc_ManageLog.vi"("Local?"="Local?", "Command"="Response", "Error In"=w12, "Refs"=w14, "Data In"=w10) -> ("Error Out"=w16:errorcluster)  [unwired: 5 in, 1 out]
    }
    frame Error {
    }
  }
  "Error Out" <- w1
